vi "sugarprice.vi"() -> (3 "Numeric":dbl)   [LabVIEW 2021]
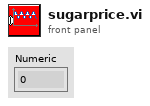
[diagram p1: front panel]
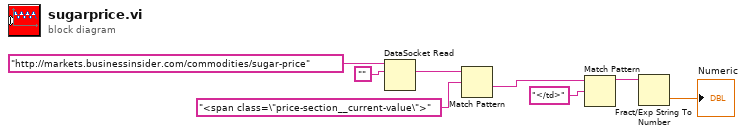
[diagram p0: block diagram]
diagram:
  n1 = DataSocket Read(10:"", 11:"http://markets.businessinsider.com/commodities/sugar-price") -> (2:w5:string)  [unwired: 3 in, 6 out]
  n2 = Match Pattern(string=w5, regular expression="<span class=\"price-section__current-value\">") -> (after substring=w3:string)  [unwired: 1 in, 3 out]
  n3 = Match Pattern(string=w3, regular expression="</td>") -> (before substring=w1:string)  [unwired: 1 in, 3 out]
  n4 = Fract/Exp String To Number(string=w1) -> (number=→"Numeric":dbl)  [unwired: 3 in, 1 out]
